vi "TeleopLogic.vi"() -> ()   [LabVIEW 2018]
uses:
  <vilib>/Rock Robotics/WPI/Relay/WPI_RelayValue.ctl
  <vilib>/Rock Robotics/WPI/Utilities/WPI_GetSetVariantRefNum.vi
  Globals.vi
panel:
  out "CancelZeroHatch":bool
  # "Copilot Controls:\nRight button: toggle arm out\nRight switch: hold down to release hatch\nLeft button: zero hatch position\nLeft switch: flip cargo out\nA button: lift low\nB button: lift mid\nY button: lift high\nRight joystick y axis: up/down front climber\nLeft joystick y axis: up/down back climber\nPOV hat up: drive forward climber wheel\nPOV hat down: drop center wheel"
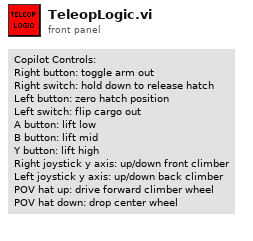
[diagram p1: front panel]
types:
  T1 = typedef "WPI_JoystickDevRef.ctl" = cluster{"Device":T2}
  T2 = typedef "WPI_JoystickDeviceEnum.ctl" = enum16{"USB 0", "USB 1", "USB 2", "USB 3", "USB 4", "USB 5"}
  T3 = typedef "WPI_RelayDevRef.ctl" = cluster{"DevStatus":errorcluster, "Relay Channel":T4, "Relay Direction":T5}
  T4 = typedef "FPGA_DIORelayChannel.ctl" = enum8{"Relay 0", "Relay 1", "Relay 2", "Relay 3", "Invalid"}
  T5 = typedef "WPI_RelayDirection.ctl" = enum16{"Both directions", "Forward only", "Reverse only"}
  T6 = typedef "WPI_RelayValue.ctl" = enum16{"Off", "On", "Forward", "Reverse"}
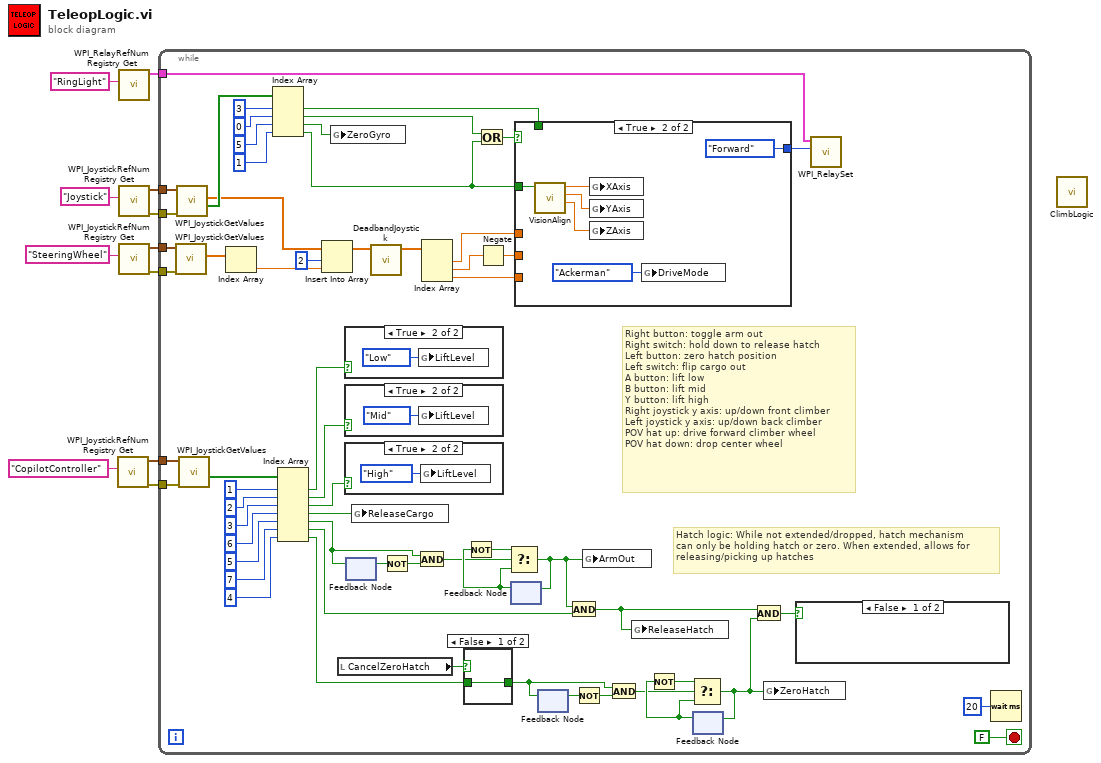
[diagram p0: block diagram]
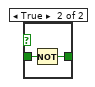
[diagram p2: hidden frame]
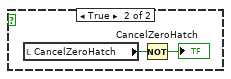
[diagram p3: hidden frame]
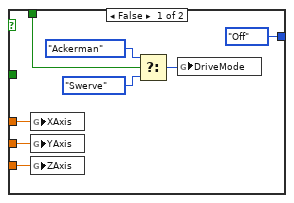
[diagram p4: hidden frame]
diagram:
  n1 = call <vilib>:"WPI_JoystickRefNum Registry Get.vi"("refnum name"="CopilotController") -> ("error out"=w4:errorcluster, "JoystickDevRef"=w6:T1)  [unwired: 1 in, 8 out]
  n2 = call <vilib>:"WPI_RelayRefNum Registry Get.vi"("refnum name"="RingLight") -> ("RelayDevRef"=w2:T3)  [unwired: 9 in, 1 out]
  n3 = call <vilib>:"WPI_JoystickRefNum Registry Get.vi"("refnum name"="Joystick") -> ("error out"=w1:errorcluster, "JoystickDevRef"=w8:T1)  [unwired: 1 in, 8 out]
  n4 = call <vilib>:"WPI_JoystickRefNum Registry Get.vi"("refnum name"="SteeringWheel") -> ("error out"=w5:errorcluster, "JoystickDevRef"=w7:T1)  [unwired: 1 in, 8 out]
  n5 = while {
    tunnel: w8 -> [w67]
    tunnel: w7 -> [w66]
    tunnel: w6 -> [w65]
    tunnel: w5 -> [w44]
    tunnel: w4 -> [w43]
    tunnel: w2 -> [w40]
    tunnel: w1 -> [w39]
    stop <- FALSE stop-if-true
    # "Hatch logic: While not extended/dropped, hatch mechanism\ncan only be holding hatch or zero. When extended, allows for\nreleasing/picking up hatches"
    # "Right button: toggle arm out\nRight switch: hold down to release hatch\nLeft button: zero hatch position\nLeft switch: flip cargo out\nA button: lift low\nB button: lift mid\nY button: lift high\nRight joystick y axis: up/down front climber\nLeft joystick y axis: up/down back climber\nPOV hat up: drive forward climber wheel\nPOV hat down: drop center wheel"
    n6 = call <vilib>:"WPI_JoystickGetValues.vi"("error in (no error)"=w44, "JoystickDevRef"=w66) -> ("Axes"=w72:dbl[])  [unwired: 5 in, 4 out]
    n7 = call <vilib>:"WPI_JoystickGetValues.vi"("error in (no error)"=w39, "JoystickDevRef"=w67) -> ("Buttons"=w71:bool[], "Axes"=w38:dbl[])  [unwired: 5 in, 3 out]
    n8 = call <vilib>:"WPI_JoystickGetValues.vi"("error in (no error)"=w43, "JoystickDevRef"=w65) -> ("Buttons"=w54:bool[])  [unwired: 5 in, 4 out]
    n9 = Index Array(array=w72) -> (element=w47:dbl)  [unwired: 1 in]
    n10 = Index Array(array=w71, index #1=3 ("index"), index #2=0 ("index"), index #3=5 ("index"), index #4=1 ("index")) -> (element #1=w34:bool, element #2=w35:bool, element #3=w46:bool, element #4=w33:bool)
    n11 = Index Array(array=w54, index #1=1 ("index"), index #2=2 ("index"), index #3=3 ("index"), index #4=6 ("index"), index #5=5 ("index"), index #6=7 ("index"), index #7=4 ("index")) -> (element #1=w59:bool, element #2=w58:bool, element #3=w57:bool, element #4=w56:bool, element #5=w16:bool, element #6=w14:bool, element #7=w22:bool)
    n12 = Insert Into Array(array=w38, index=2, new element=w47) -> (w48:dbl[])
    n13 = global write "Globals.vi" "ZeroGyro"(w46) -> ()
    n14 = local read "CancelZeroHatch"() -> (w31:bool)
    n15 = case shown="True" w59 {
      frame False {
      }
      frame True {
        n16 = global write "Globals.vi" "LiftLevel"(enum16{"Low", "Mid", "High"}."Low" ("LiftLevel")) -> ()
      }
    }
    n17 = case shown="True" w58 {
      frame False {
      }
      frame True {
        n18 = global write "Globals.vi" "LiftLevel"(enum16{"Low", "Mid", "High"}."Mid" ("LiftLevel")) -> ()
      }
    }
    n19 = case shown="True" w57 {
      frame False {
      }
      frame True {
        n20 = global write "Globals.vi" "LiftLevel"(enum16{"Low", "Mid", "High"}."High" ("LiftLevel")) -> ()
      }
    }
    n21 = feedback #1() -> (w17:bool)  [unwired: 1 in]
    n22 = feedback-in #1(w16) -> ()
    n23 = global write "Globals.vi" "ReleaseCargo"(w56) -> ()
    n24 = call "DeadbandJoystick.vi"("InputArray"=w48) -> ("OutputArray"=w53:dbl[])  [unwired: 10 in]
    n25 = Not(x=w17) -> (.not. x?=w18:bool)
    n26 = And(x=w16, y=w18) -> (x .and. y?=w19:bool)
    n27 = Index Array(array=w53) -> (element #1=w45:dbl, element #2=w52:dbl, element #3=w51:dbl)  [unwired: 3 in]
    n28 = case shown="False" w31 {
      tunnel: [w73 w74] -> w25
      tunnel: w22 -> [w73 w75]
      frame False {
      }
      frame True {
        n29 = Not(x=w75) -> (.not. x?=w74:bool)
      }
    }
    n30 = Or(x=w35, y=w33) -> (x .or. y?=w36:bool)
    n31 = Negate(x=w52) -> (-x=w50:dbl)
    n32 = feedback #2() -> (w20:bool)  [unwired: 1 in]
    n33 = Not(x=w20) -> (.not. x?=w21:bool)
    n34 = Select(t=w21, s=w19, f=w20) -> (s? t:f=w15:bool)
    n35 = feedback-in #2(w15) -> ()
    n36 = case shown="True" w36 {
      tunnel: w51 -> [w84 _]
      tunnel: w50 -> [w85 _]
      tunnel: w45 -> [w81 _]
      tunnel: [WPI_RelayValue."Off" ("RelayValue") WPI_RelayValue."Forward" ("RelayValue")] -> w41
      tunnel: w33 -> [_ w88]
      tunnel: w34 -> [w83 _]
      frame False {
        n37 = global write "Globals.vi" "XAxis"(w81) -> ()
        n38 = global write "Globals.vi" "YAxis"(w85) -> ()
        n39 = global write "Globals.vi" "ZAxis"(w84) -> ()
        n40 = Select(t=enum16{"Swerve", "Ackerman"}."Ackerman" ("DriveMode"), s=w83, f=enum16{"Swerve", "Ackerman"}."Swerve") -> (s? t:f=w82:enum16{"Swerve", "Ackerman"})
        n41 = global write "Globals.vi" "DriveMode"(w82) -> ()
      }
      frame True {
        n42 = call "VisionAlign.vi"("CargoShipAlign"=w88) -> ("Z"=w91:dbl, "Y"=w87:dbl, "X"=w90:dbl)  [unwired: 8 in]
        n43 = global write "Globals.vi" "XAxis"(w90) -> ()
        n44 = global write "Globals.vi" "YAxis"(w87) -> ()
        n45 = global write "Globals.vi" "ZAxis"(w91) -> ()
        n46 = global write "Globals.vi" "DriveMode"(enum16{"Swerve", "Ackerman"}."Ackerman" ("DriveMode")) -> ()
      }
    }
    n47 = feedback #3() -> (w26:bool)  [unwired: 1 in]
    n48 = feedback-in #3(w25) -> ()
    n49 = And(x=w15, y=w14) -> (x .and. y?=w13:bool)
    n50 = Not(x=w26) -> (.not. x?=w27:bool)
    n51 = global write "Globals.vi" "ArmOut"(w15) -> ()
    n52 = And(x=w25, y=w27) -> (x .and. y?=w28:bool)
    n53 = global write "Globals.vi" "ReleaseHatch"(w13) -> ()
    n54 = feedback #4() -> (w29:bool)  [unwired: 1 in]
    n55 = Not(x=w29) -> (.not. x?=w30:bool)
    n56 = Select(t=w30, s=w28, f=w29) -> (s? t:f=w23:bool)
    n57 = feedback-in #4(w23) -> ()
    n58 = And(x=w13, y=w23) -> (x .and. y?=w24:bool)
    n59 = global write "Globals.vi" "ZeroHatch"(w23) -> ()
    n60 = case shown="False" w24 {
      frame False {
      }
      frame True {
        n61 = local read "CancelZeroHatch"() -> (w77:bool)
        n62 = Not(x=w77) -> (.not. x?=→"CancelZeroHatch":bool)
      }
    }
    n63 = call <vilib>:"WPI_RelaySet.vi"("RelayValue"=w41, "RelayDevRef"=w40) -> ()  [unwired: 8 in, 2 out]
    n64 = Wait (ms)(milliseconds to wait=u32 20) -> ()  [unwired: 1 out]
  }
  n65 = call "ClimbLogic.vi"() -> ()  [unwired: 12 in]
